vi "Accelerate.vi"(10 "Direction":T1, 11 "Snake in":refnum<class "Snake.lvclass">) -> (3 "Snake out":refnum<class "Snake.lvclass">)   [LabVIEW 2020, in "Snake.lvclass"]
uses:
  Snake.lvclass
  Direction.ctl
  Snake.lvclass/Snake.ctl
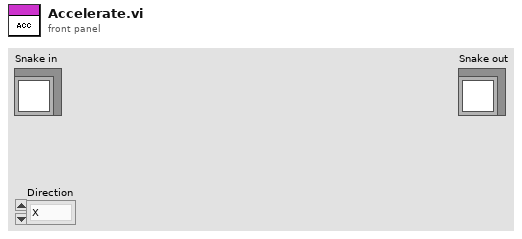
[diagram p1: front panel]
types:
  T1 = typedef "Direction.ctl" = enum16{"X", "-X", "Y", "-Y"}
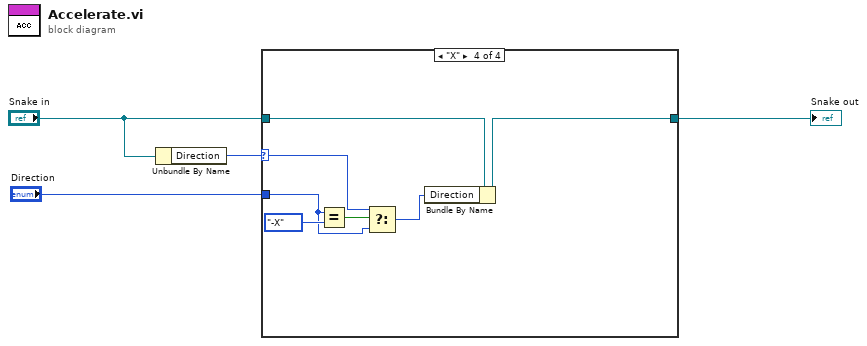
[diagram p0: block diagram]
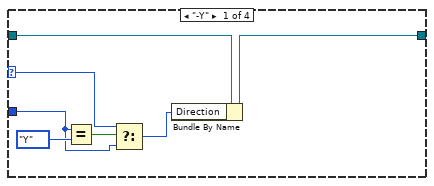
[diagram p2: hidden frame]
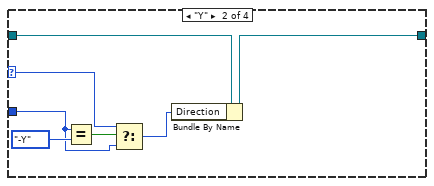
[diagram p3: hidden frame]
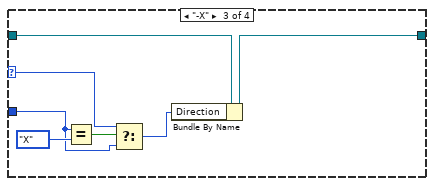
[diagram p4: hidden frame]
diagram:
  n1 = Unbundle By Name("Snake in") -> ("Direction"=w1:T1)
  n2 = case shown="\"X\"" w1 {
    selector: w1 -> [w8 w15 w22 w29]
    tunnel: [w11 w18 w25 w32] -> w4
    tunnel: "Direction" -> [w6 w13 w20 w27]
    tunnel: "Snake in" -> [w10 w17 w24 w31]
    frame "-Y" {
      n3 = Equal?(x=w6, y=Direction."Y") -> (x = y?=w7:bool)
      n4 = Select(t=w8, s=w7, f=w6) -> (s? t:f=w5:T1)
      n5 = Bundle By Name(cluster=w10, "Direction"=w5) -> (w11:refnum<class "Snake.lvclass">)
    }
    frame "Y" {
      n6 = Equal?(x=w13, y=Direction."-Y") -> (x = y?=w14:bool)
      n7 = Select(t=w15, s=w14, f=w13) -> (s? t:f=w12:T1)
      n8 = Bundle By Name(cluster=w17, "Direction"=w12) -> (w18:refnum<class "Snake.lvclass">)
    }
    frame "-X" {
      n9 = Equal?(x=w20, y=Direction."X") -> (x = y?=w21:bool)
      n10 = Select(t=w22, s=w21, f=w20) -> (s? t:f=w19:T1)
      n11 = Bundle By Name(cluster=w24, "Direction"=w19) -> (w25:refnum<class "Snake.lvclass">)
    }
    frame "X" {
      n12 = Equal?(x=w27, y=Direction."-X") -> (x = y?=w28:bool)
      n13 = Select(t=w29, s=w28, f=w27) -> (s? t:f=w26:T1)
      n14 = Bundle By Name(cluster=w31, "Direction"=w26) -> (w32:refnum<class "Snake.lvclass">)
    }
  }
  "Snake out" <- w4
